vi "Integrate.vi"(9 "Elapsed Sec":dbl, 11 "Rate":dbl) -> (3 "DIST":dbl)   [LabVIEW 2019]
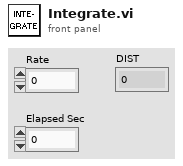
[diagram p1: front panel]
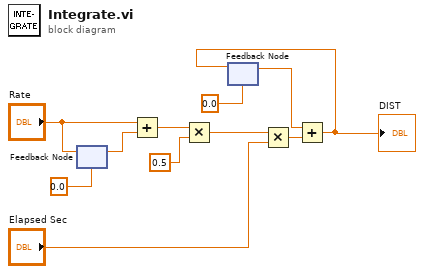
[diagram p0: block diagram]
diagram:
  n1 = feedback #1(0.0 ("Rate")) -> (w6:dbl)
  n2 = feedback-in #1("Rate") -> ()
  n3 = Add(x="Rate", y=w6) -> (x+y=w4:dbl)
  n4 = Multiply(x=w4, y=0.5) -> (x*y=w1:dbl)
  n5 = feedback #2(0.0 ("Rate")) -> (w10:dbl)
  n6 = Multiply(x=w1, y="Elapsed Sec") -> (x*y=w9:dbl)
  n7 = Add(x=w10, y=w9) -> (x+y=w11:dbl)
  "DIST" <- w11
  n8 = feedback-in #2(w11) -> ()
